vi "uEye_SimpleLive.vi"() -> ()   [LabVIEW 2016]
uses:
  C:/Program Files/National Instruments/LabVIEW 2016/instr.lib/IDS/ueye.NET/uEyeDotNet.dll
  Program Files/National Instruments/LabVIEW 2016/instr.lib/IDS/ueye.NET/uEyeDotNet.dll
  System.Windows.Forms
panel:
  in  "Exposure":dbl(slide) min=0.07826829268292683 max=49.96831707317074 step=0.021121951219512197 scale=0.0769533433340476..166.26649730429713
  out "MinFps":i32=8
  out "MaxFps":i32=8
  in  "Framerate":dbl min=3.056022538005872 max=6.160183642413259 step=0.0031285848869551103
  in  "Pixelclock":u16(ring) items=["5", "6", "7", "8", "9", "10", "11", "12", "13", "14", "15", "16", "17", "18", "19", "20", "21", "22", "23", "24", "25", "26", "27", "28", "29", "30", "31", "32", "33", "34", "35", "36", "37", "38", "39", "40", "41", "42"]
  in  "Auto Exposure":bool
  in  "Zoom":u16(ring)=1 items=["4X"=4, "2X"=2, "1X"=1]
  in  "PictureBox":refnum<k24>(container)
  out "Serial Number 2":string
  out "Height 2":i32=8
  out "Width 2":i32=8
  out "Bits/Pixel 2":i32=8
  in  "Camera ID":i32
  out "Serial Number":string
  out "Height":i32=8
  out "Width":i32=8
  out "Bits/Pixel":i32=8
  out "Error Out":errorcluster caption="error"
  in  "Load Parameter":bool
  in  "Exit Camera":bool
  in  "Stop Live":bool
  in  "Start Live":bool
  in  "Init Camera":bool
  # "-"
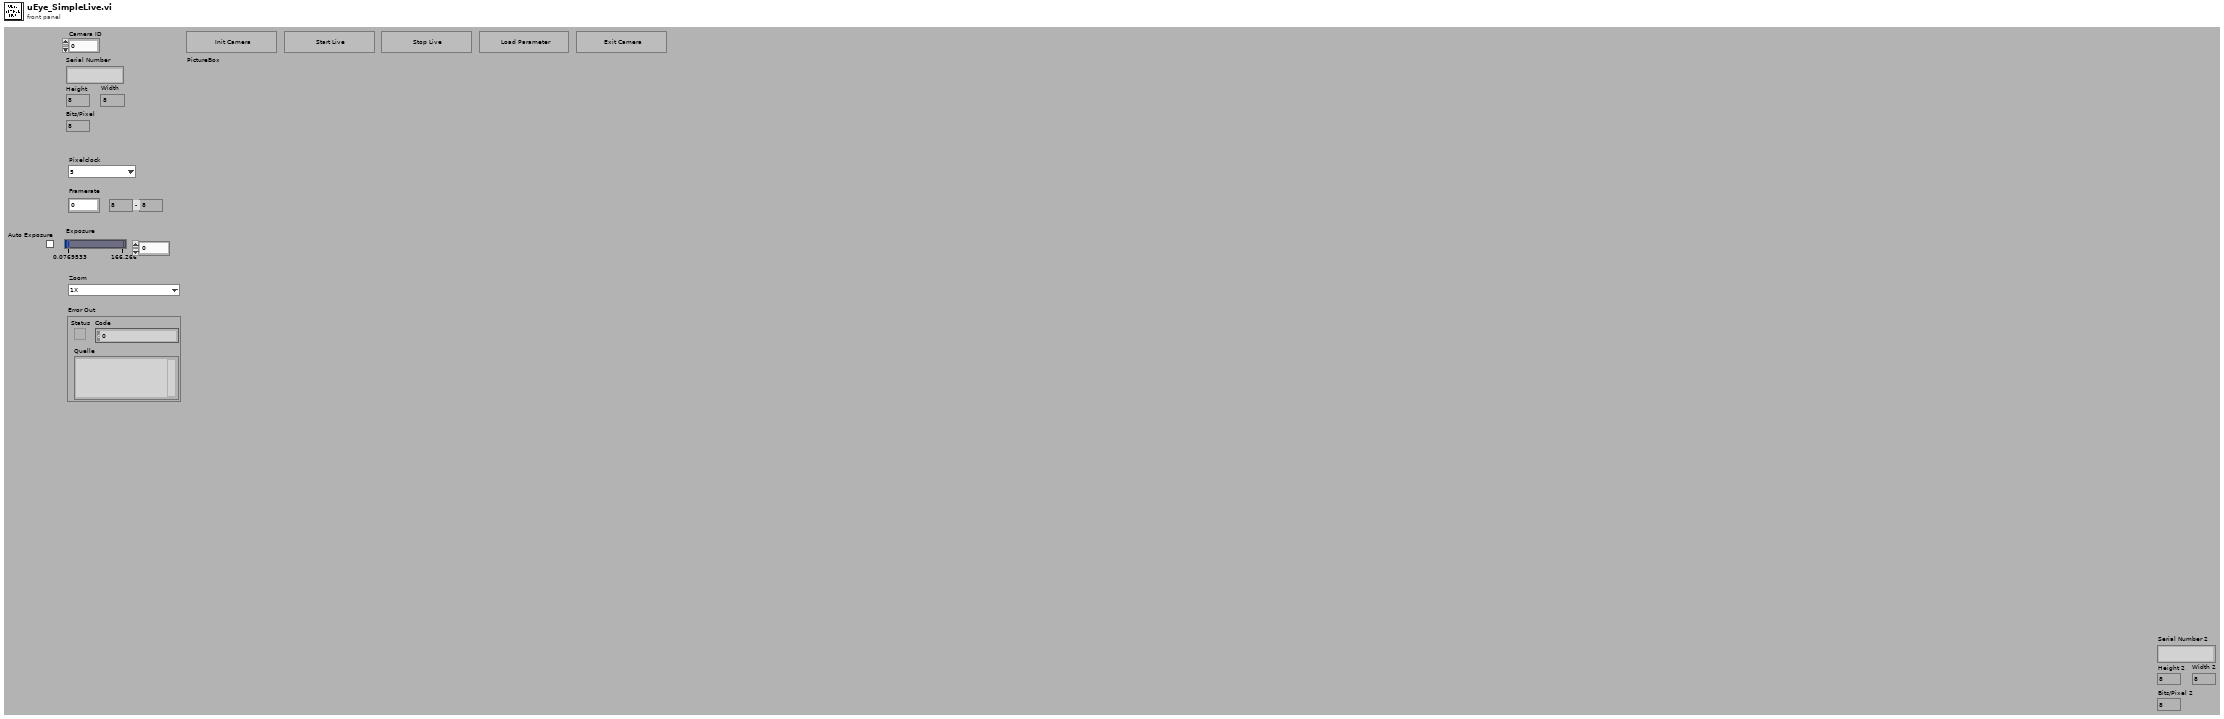
[diagram p1: front panel]
types:
  T1 = enum8{"Enabled", "Disabled", "Disabled and Grayed Out"}
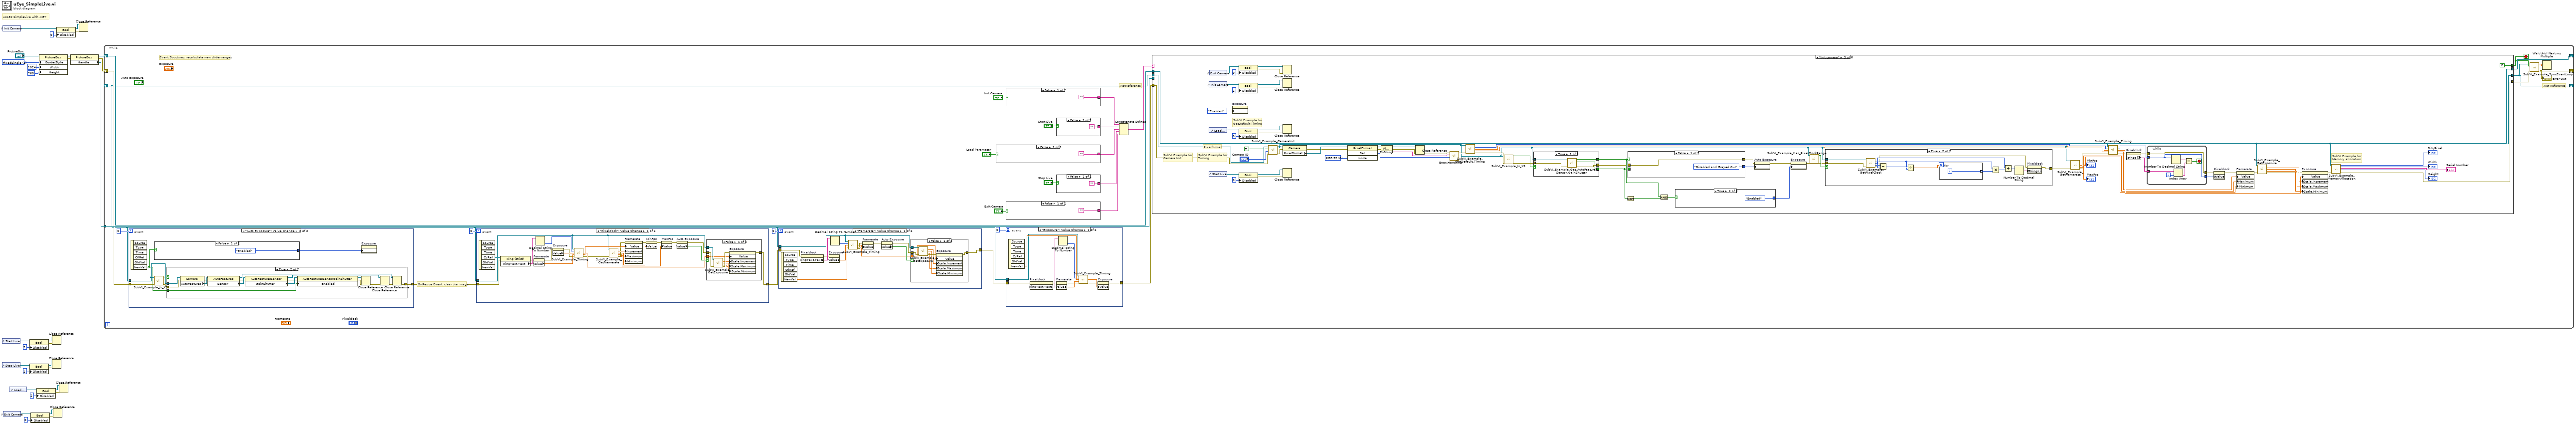
[diagram p0: block diagram]
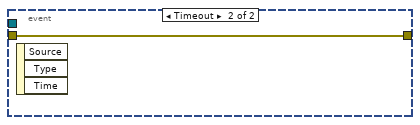
[diagram p2: hidden frame]
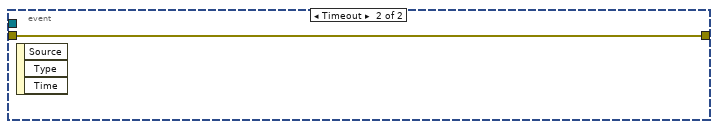
[diagram p4: hidden frame]
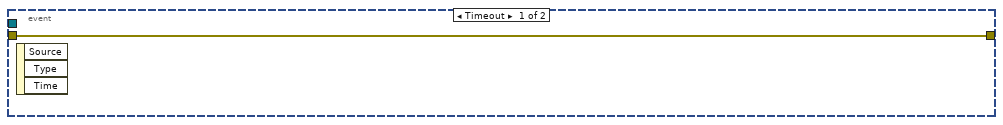
[diagram p5: hidden frame]
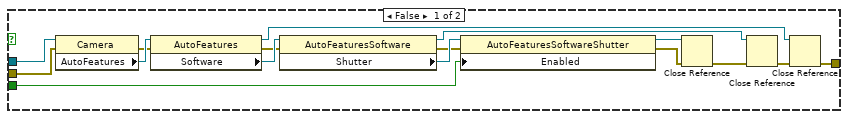
[diagram p6: hidden frame]
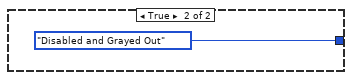
[diagram p7: hidden frame]
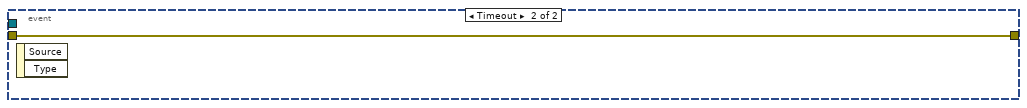
[diagram p9: hidden frame]
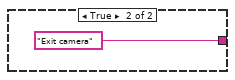
[diagram p10: hidden frame]
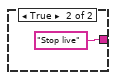
[diagram p11: hidden frame]
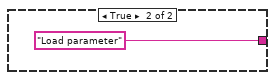
[diagram p12: hidden frame]
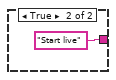
[diagram p13: hidden frame]
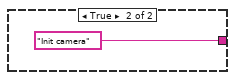
[diagram p14: hidden frame]
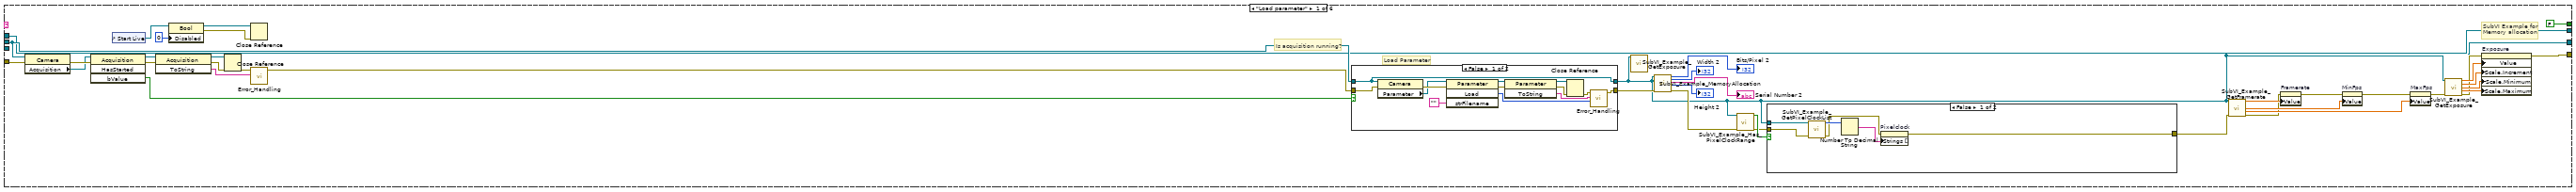
[diagram p15: hidden frame]
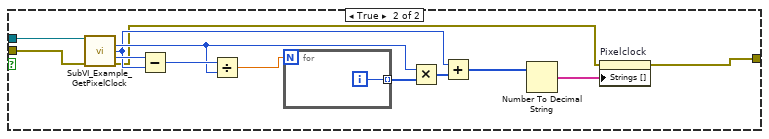
[diagram p16: hidden frame]
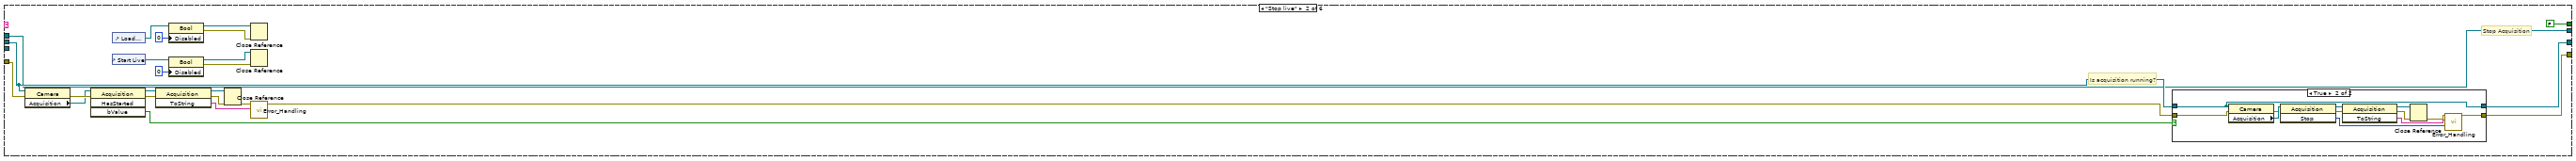
[diagram p18: hidden frame]
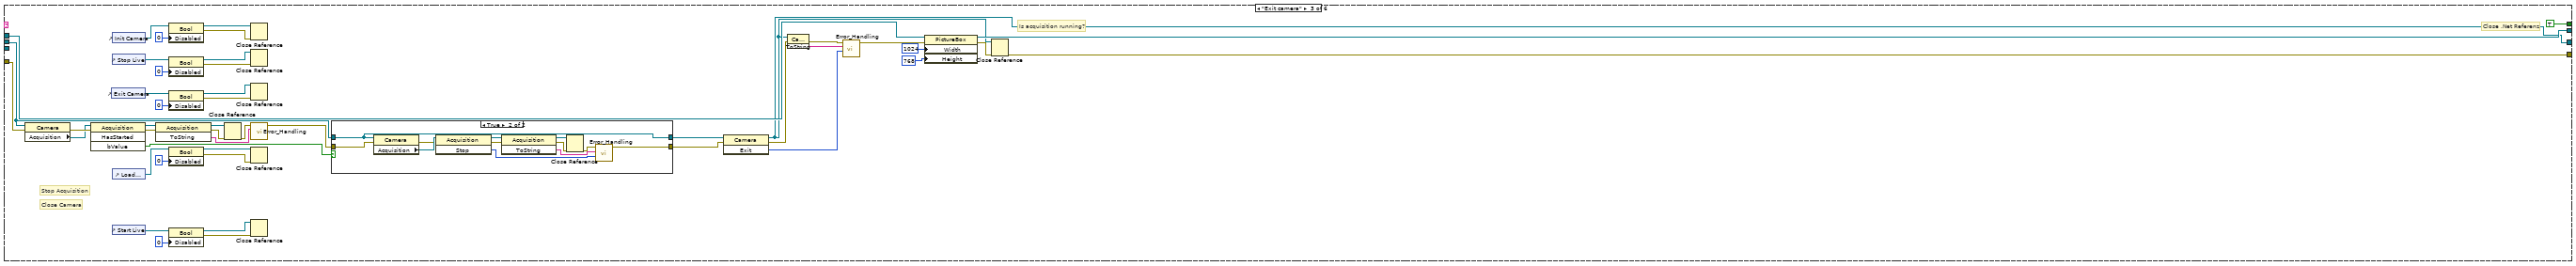
[diagram p20: hidden frame]
diagram:
  w18 = 1 items=["None", "FixedSingle", "Fixed3D"] ("BorderStyle")
  # "uc480 SimpleLive with .NET"
  n1 = control-ref of="Start Live"() -> (w26:refnum<vi>)
  n2 = control-ref of="Stop Live"() -> (w20:refnum<vi>)
  n3 = control-ref of="Init Camera"() -> (w29:refnum<vi>)
  n4 = control-ref of="Exit Camera"() -> (w22:refnum<vi>)
  n5 = control-ref of="Load Parameter"() -> (w21:refnum<vi>)
  n6 = property class="Bool"(reference=w26, "Disabled"=u8 2 ("Deaktiviert")) -> (reference out=w13:refnum<vi>, error out=w12:errorcluster)  [unwired: 1 in]
  n7 = property class="Bool"(reference=w20, "Disabled"=u8 2 ("Deaktiviert")) -> (reference out=w11:refnum<vi>, error out=w10:errorcluster)  [unwired: 1 in]
  n8 = property class="Bool"(reference=w22, "Disabled"=u8 0 ("Deaktiviert")) -> (reference out=w7:refnum<vi>, error out=w6:errorcluster)  [unwired: 1 in]
  n9 = property class="Bool"(reference=w21, "Disabled"=u8 2 ("Deaktiviert")) -> (reference out=w9:refnum<vi>, error out=w8:errorcluster)  [unwired: 1 in]
  n10 = property class="PictureBox"(reference="PictureBox", "BorderStyle"=w18, "Width"=1024, "Height"=768) -> (reference out=w4:refnum<k24>, error out=w5:errorcluster)  [unwired: 1 in]
  n11 = Close Reference(reference=w13, error in (no error)=w12) -> ()  [unwired: 1 out]
  n12 = Close Reference(reference=w11, error in (no error)=w10) -> ()  [unwired: 1 out]
  n13 = Close Reference(reference=w7, error in (no error)=w6) -> ()  [unwired: 1 out]
  n14 = property class="Bool"(reference=w29, "Disabled"=u8 0 ("Deaktiviert")) -> (reference out=w15:refnum<vi>, error out=w14:errorcluster)  [unwired: 1 in]
  n15 = Close Reference(reference=w9, error in (no error)=w8) -> ()  [unwired: 1 out]
  n16 = property class="PictureBox"(reference=w4, error in=w5) -> (reference out=w3:refnum<k24>, error out=w2:errorcluster, "Handle"=w1:refnum<k24>)
  n17 = Close Reference(reference=w15, error in (no error)=w14) -> ()  [unwired: 1 out]
  n18 = while {
    shift-right: [w45] -> _
    shift-left: w2 -> [w41]
    shift-right: [w30] -> _
    shift-left: _ -> [w35]
    shift-right: [w44] -> _
    shift-left: w3 -> [w40]
    tunnel: w1 -> [w43]
    stop <- w31 stop-if-true
    # "OnResize Event, clear the image"
    # "Event Structures, recalculate new slider ranges"
    # ".NetReference"
    # ".Net Reference"
    n19 = event shown="[1] \"Auto Exposure\": Value Change" {
      selector: _ -> [_ _]
      dyn-events: _ -> [_ _]
      timeout: 0 -> [_ _]
      tunnel: w41 -> [w95 w102]
      tunnel: w35 -> [_ w100]
      tunnel: [w95 w97] -> w39
      event Timeout {
        n20 = event-data() -> ()  [unwired: 1 in, 3 out]
      }
      event "Auto Exposure": Value Change {
        n21 = event-data() -> ("NewVal"=w99:bool)  [unwired: 1 in, 5 out]
        n22 = case shown="False" w99 {
          tunnel: [T1."Enabled" ("Deaktiviert") T1."Disabled and Grayed Out" ("Deaktiviert")] -> w96
          frame False {
          }
          frame True {
          }
        }
        n23 = call "SubVI_Example_Is_XS.vi"("Error In"=w102, ".NET (Reference)"=w100) -> ("Error Out"=w101:errorcluster, "IsXS"=w98:bool)  [unwired: 7 in, 1 out]
        n24 = case shown="True" w98 {
          tunnel: w101 -> [w106 w133]
          tunnel: [w103 w119] -> w97
          tunnel: w100 -> [w105 w134]
          tunnel: w99 -> [w104 w126]
          frame False {
            n25 = property on="Eigenschaftsknoten" class="Camera"(reference=w105, error in=w106) -> (error out=w117:errorcluster, "AutoFeatures"=w118:refnum<k24>)  [unwired: 1 out]
            n26 = property on="Eigenschaftsknoten" class="AutoFeatures"(reference=w118, error in=w117) -> (reference out=w107:refnum<k24>, error out=w115:errorcluster, "Software"=w116:refnum<k24>)
            n27 = property on="Eigenschaftsknoten" class="AutoFeaturesSoftware"(reference=w116, error in=w115) -> (reference out=w110:refnum<k24>, error out=w113:errorcluster, "Shutter"=w114:refnum<k24>)
            n28 = property on="Eigenschaftsknoten" class="AutoFeaturesSoftwareShutter"(reference=w114, error in=w113, "Enabled"=w104) -> (reference out=w112:refnum<k24>, error out=w111:errorcluster)
            n29 = Close Reference(reference=w112, error in (no error)=w111) -> (error out=w109:errorcluster)
            n30 = Close Reference(reference=w110, error in (no error)=w109) -> (error out=w108:errorcluster)
            n31 = Close Reference(reference=w107, error in (no error)=w108) -> (error out=w103:errorcluster)
          }
          frame True {
            n32 = property on="Eigenschaftsknoten" class="Camera"(reference=w134, error in=w133) -> (error out=w131:errorcluster, "AutoFeatures"=w132:refnum<k24>)  [unwired: 1 out]
            n33 = property on="Eigenschaftsknoten" class="AutoFeatures"(reference=w132, error in=w131) -> (reference out=w120:refnum<k24>, error out=w129:errorcluster, "Sensor"=w130:refnum<k24>)
            n34 = property on="Eigenschaftsknoten" class="AutoFeaturesSensor"(reference=w130, error in=w129) -> (reference out=w123:refnum<k24>, error out=w127:errorcluster, "GainShutter"=w128:refnum<k24>)
            n35 = property on="Eigenschaftsknoten" class="AutoFeaturesSensorGainShutter"(reference=w128, error in=w127, "Enabled"=w126) -> (reference out=w125:refnum<k24>, error out=w124:errorcluster)
            n36 = Close Reference(reference=w125, error in (no error)=w124) -> (error out=w122:errorcluster)
            n37 = Close Reference(reference=w123, error in (no error)=w122) -> (error out=w121:errorcluster)
            n38 = Close Reference(reference=w120, error in (no error)=w121) -> (error out=w119:errorcluster)
          }
        }
        n39 = property on="Exposure" class="Slide (strict)"("DisabledEnum"=w96) -> ()  [unwired: 2 in, 2 out]
      }
    }
    n40 = event shown="[0] \"Pixelclock\": Value Change" {
      selector: _ -> [_ _]
      dyn-events: _ -> [_ _]
      timeout: 0 -> [_ _]
      tunnel: w35 -> [w149 _]
      tunnel: w39 -> [w141 w169]
      tunnel: [w146 w169] -> w38
      event "Pixelclock": Value Change {
        n41 = event-data() -> ("CtlRef"=w144:refnum<vi>)  [unwired: 1 in, 5 out]
        n42 = property class="Ring (strict)"(reference=w144, error in=w141) -> (error out=w140:errorcluster, "RingText.Text"=w143:string)  [unwired: 1 out]
        n43 = property on="Framerate" class="DigNum (strict)"(error in=w140) -> (error out=w139:errorcluster, "Value"=w159:dbl)  [unwired: 1 in, 1 out]
        n44 = Decimal String To Number(string=w143) -> (number=w142:i32)  [unwired: 2 in, 1 out]
        n45 = property on="Exposure" class="Slide (strict)"(error in=w139) -> (error out=w138:errorcluster, "Value"=w158:dbl)  [unwired: 1 in, 1 out]
        n46 = call "SubVI_Example_Timing.vi"(".NET (Reference)"=w149, "Pixelclock"=w142, "Exposure time"=w158, "Framerate"=w159, "Error In"=w138) -> ("Exposure time"=w145:dbl, "Framerate"=w156:dbl, "Error Out"=w137:errorcluster)  [unwired: 7 in, 1 out]
        n47 = call "SubVI_Example_GetFramerate.vi"(".NET (Reference)"=w149, "Error In"=w137) -> ("Inc"=w157:dbl, "Min"=w154:dbl, "Max"=w153:dbl, "error out"=w155:errorcluster)  [unwired: 9 in, 1 out]
        n48 = property on="Framerate" class="DigNum (strict)"(error in=w155, "Value"=w156, "Increment"=w157, "Maximum"=w153, "Minimum"=w154) -> (error out=w152:errorcluster)  [unwired: 1 in, 1 out]
        n49 = property on="MinFps" class="DigNum (strict)"(error in=w152, "Value"=w154) -> (error out=w151:errorcluster)  [unwired: 1 in, 1 out]
        n50 = property on="MaxFps" class="DigNum (strict)"(error in=w151, "Value"=w153) -> (error out=w148:errorcluster)  [unwired: 1 in, 1 out]
        n51 = property on="Auto Exposure" class="Bool (strict)"(error in=w148) -> (error out=w147:errorcluster, "Value"=w150:bool)  [unwired: 1 in, 1 out]
        n52 = case shown="False" w150 {
          tunnel: w149 -> [w167 _]
          tunnel: w147 -> [w166 w168]
          tunnel: [w164 w168] -> w146
          tunnel: w145 -> [w160 _]
          frame False {
            n53 = call "SubVI_Example_GetExposure.vi"(".NET (Reference)"=w167, "Error In"=w166) -> ("Inc"=w161:dbl, "Min"=w163:dbl, "Max"=w162:dbl, "Error out"=w165:errorcluster)  [unwired: 9 in, 1 out]
            n54 = property on="Exposure" class="Slide (strict)"(error in=w165, "Value"=w160, "Scale.Increment"=w161, "Scale.Maximum"=w162, "Scale.Minimum"=w163) -> (error out=w164:errorcluster)  [unwired: 1 in, 1 out]
          }
          frame True {
          }
        }
      }
      event Timeout {
        n55 = event-data() -> ()  [unwired: 1 in, 2 out]
      }
    }
    n56 = event shown="[0] \"Framerate\": Value Change" {
      selector: _ -> [_ _]
      dyn-events: _ -> [_ _]
      timeout: 0 -> [_ _]
      tunnel: w38 -> [w72 w94]
      tunnel: w35 -> [w76 _]
      tunnel: [w77 w94] -> w34
      event "Framerate": Value Change {
        n57 = event-data() -> ("NewVal"=w84:dbl)  [unwired: 1 in, 5 out]
        n58 = property on="Pixelclock" class="Ring (strict)"(error in=w72) -> (error out=w71:errorcluster, "RingText.Text"=w74:string)  [unwired: 1 in, 1 out]
        n59 = property on="Exposure" class="Slide (strict)"(error in=w71) -> ("Value"=w83:dbl)  [unwired: 1 in, 2 out]
        n60 = Decimal String To Number(string=w74) -> (number=w73:i32)  [unwired: 2 in, 1 out]
        n61 = call "SubVI_Example_Timing.vi"(".NET (Reference)"=w76, "Pixelclock"=w73, "Exposure time"=w83, "Framerate"=w84) -> ("Exposure time"=w75:dbl, "Framerate"=w82:dbl, "Error Out"=w80:errorcluster)  [unwired: 8 in, 1 out]
        n62 = property on="Framerate" class="DigNum (strict)"(error in=w80, "Value"=w82) -> (error out=w79:errorcluster)  [unwired: 1 in, 1 out]
        n63 = property on="Auto Exposure" class="Bool (strict)"(error in=w79) -> (error out=w78:errorcluster, "Value"=w81:bool)  [unwired: 1 in, 1 out]
        n64 = case shown="False" w81 {
          tunnel: w78 -> [w92 w93]
          tunnel: [w90 w93] -> w77
          tunnel: w76 -> [w89 _]
          tunnel: w75 -> [w85 _]
          frame False {
            n65 = call "SubVI_Example_GetExposure.vi"(".NET (Reference)"=w89, "Error In"=w92) -> ("Inc"=w87:dbl, "Min"=w88:dbl, "Max"=w86:dbl, "Error out"=w91:errorcluster)  [unwired: 9 in, 1 out]
            n66 = property on="Exposure" class="Slide (strict)"(error in=w91, "Value"=w85, "Scale.Increment"=w87, "Scale.Maximum"=w86, "Scale.Minimum"=w88) -> (error out=w90:errorcluster)  [unwired: 1 in, 1 out]
          }
          frame True {
          }
        }
      }
      event Timeout {
        n67 = event-data() -> ()  [unwired: 1 in, 3 out]
      }
    }
    n68 = case shown="False" "Load Parameter" {
      tunnel: ["" "Load parameter"] -> w52
      frame False {
      }
      frame True {
      }
    }
    n69 = case shown="False" "Init Camera" {
      tunnel: ["" "Init camera"] -> w56
      frame False {
      }
      frame True {
      }
    }
    n70 = case shown="False" "Exit Camera" {
      tunnel: ["" "Exit camera"] -> w48
      frame False {
      }
      frame True {
      }
    }
    n71 = event shown="[0] \"Exposure\": Value Change" {
      selector: _ -> [_ _]
      dyn-events: _ -> [_ _]
      timeout: 0 -> [_ _]
      tunnel: w35 -> [w65 _]
      tunnel: w34 -> [w61 w70]
      tunnel: [w66 w70] -> w33
      event "Exposure": Value Change {
        n72 = event-data() -> ("NewVal"=w69:dbl)  [unwired: 1 in, 5 out]
        n73 = property on="Pixelclock" class="Ring (strict)"(error in=w61) -> (error out=w60:errorcluster, "RingText.Text"=w63:string)  [unwired: 1 in, 1 out]
        n74 = property on="Framerate" class="DigNum (strict)"(error in=w60) -> (error out=w59:errorcluster, "Value"=w68:dbl)  [unwired: 1 in, 1 out]
        n75 = Decimal String To Number(string=w63) -> (number=w62:i32)  [unwired: 2 in, 1 out]
        n76 = call "SubVI_Example_Timing.vi"(".NET (Reference)"=w65, "Pixelclock"=w62, "Exposure time"=w69, "Framerate"=w68, "Error In"=w59) -> ("Exposure time"=w67:dbl, "Error Out"=w64:errorcluster)  [unwired: 7 in, 2 out]
        n77 = property on="Exposure" class="Slide (strict)"(error in=w64, "Value"=w67) -> (error out=w66:errorcluster)  [unwired: 1 in, 1 out]
      }
      event Timeout {
        n78 = event-data() -> ()  [unwired: 1 in, 3 out]
      }
    }
    n79 = case shown="False" "Start Live" {
      tunnel: ["" "Start live"] -> w55
      frame False {
      }
      frame True {
      }
    }
    n80 = case shown="False" "Stop Live" {
      tunnel: ["" "Stop live"] -> w51
      frame False {
      }
      frame True {
      }
    }
    n81 = Concatenate Strings(w56, w55, w52, w51, w48) -> (w54:string)
    n82 = case shown="\"Init camera\"" w54 {
      tunnel: w35 -> [w211 w271 w326 w360 w482 w552]
      tunnel: w33 -> [w214 w272 w327 w361 w481 w553]
      tunnel: [w181 w270 w335 w358 w451 w550] -> w47
      tunnel: [FALSE FALSE TRUE FALSE FALSE FALSE] -> w31
      tunnel: w40 -> [w203 w264 w306 w366 w463 w543]
      tunnel: [w203 w264 w305 w365 w463 w543] -> w44
      tunnel: w43 -> [_ _ _ w362 _ _]
      tunnel: [w180 w256 w294 w355 w420 w536] -> w30
      frame "Load parameter" {
        # "SubVI Example for \nMemory allocation"
        # "Is acquisition running?"
        # "Load Parameter"
        n83 = property class="Camera"(reference=w211, error in=w214) -> (error out=w219:errorcluster, "Acquisition"=w218:refnum<k24>)  [unwired: 1 out]
        n84 = invoke class="Acquisition" method="HasStarted"(reference=w218, error in=w219) -> (reference out=w215:refnum<k24>, error out=w217:errorcluster, "bValue"=w213:bool)  [unwired: 2 in, 1 out]
        n85 = control-ref of="Start Live"() -> (w205:refnum<vi>)
        n86 = invoke class="Acquisition" method="ToString"(reference=w215, error in=w217) -> (reference out=w200:refnum<k24>, error out=w199:errorcluster, "ToString"=w216:string)  [unwired: 1 in]
        n87 = property class="Bool"(reference=w205, "Disabled"=u8 0 ("Deaktiviert")) -> (reference out=w202:refnum<vi>, error out=w201:errorcluster)  [unwired: 1 in]
        n88 = Close Reference(reference=w200, error in (no error)=w199) -> (error out=w198:errorcluster)
        n89 = Close Reference(reference=w202, error in (no error)=w201) -> ()  [unwired: 1 out]
        n90 = call "Error_Handling.vi"("Error String"=w216, "Error In"=w198) -> ("Error Out"=w212:errorcluster)  [unwired: 9 in]
        n91 = case shown="False" w213 {
          tunnel: w212 -> [w247 w254]
          tunnel: w211 -> [w245 w255]
          tunnel: [w246 w254] -> w206
          tunnel: [w245 w255] -> w180
          frame False {
            n92 = property class="Camera"(reference=w245, error in=w247) -> (error out=w249:errorcluster, "Parameter"=w248:refnum<k24>)  [unwired: 1 out]
            n93 = invoke class="Parameter" method="Load"(reference=w248, error in=w249, "strFilename"="") -> (reference out=w251:refnum<k24>, error out=w252:errorcluster, "Load"=w244:i32)  [unwired: 1 in, 1 out]
            n94 = invoke class="Parameter" method="ToString"(reference=w251, error in=w252) -> (reference out=w241:refnum<k24>, error out=w243:errorcluster, "ToString"=w253:string)  [unwired: 1 in]
            n95 = Close Reference(reference=w241, error in (no error)=w243) -> (error out=w242:errorcluster)
            n96 = call "Error_Handling.vi"("Error Code"=w244, "Error String"=w253, "Error In"=w242) -> ("Error Out"=w246:errorcluster)  [unwired: 8 in]
          }
          frame True {
          }
        }
        n97 = call "SubVI_Example_GetExposure.vi"(".NET (Reference)"=w180) -> ()  [unwired: 10 in, 5 out]
        n98 = call "SubVI_Example_MemoryAllocation.vi"(".NET (Reference)"=w180, "Error In"=w206) -> ("Bits/Pixel 2"=→"Bits/Pixel 2":i32, "Width"=→"Width 2":i32, "Serial Number"=→"Serial Number 2":string, "Height"=→"Height 2":i32, "Error Out"=w197:errorcluster)  [unwired: 13 in]
        n99 = call "SubVI_Example_Has_PixelClockRange.vi"(".NET (Reference)"=w180, "error in (no error)"=w197) -> ("Boolean"=w196:bool, "error out"=w195:errorcluster)  [unwired: 16 in]
        n100 = case shown="False" w196 {
          tunnel: w195 -> [w226 w239]
          tunnel: w180 -> [w225 w238]
          tunnel: [w221 w227] -> w194
          frame False {
            n101 = call "SubVI_Example_GetPixelClockList.vi"("error in (no error)"=w226, ".NET (Reference)"=w225) -> ("error out"=w222:errorcluster, "List"=w224:i32[])  [unwired: 7 in, 1 out]
            n102 = Number To Decimal String(number=w224) -> (decimal integer string=w223:string[])  [unwired: 1 in]
            n103 = property on="Pixelclock" class="Ring (strict)"(error in=w222, "Strings []"=w223) -> (error out=w221:errorcluster)  [unwired: 1 in, 1 out]
          }
          frame True {
            n104 = call "SubVI_Example_GetPixelClock.vi"(".NET (Reference)"=w238, "Error In"=w239) -> ("Inc"=w233:i32, "Min"=w231:i32, "Max"=w237:i32, "error out"=w228:errorcluster)  [unwired: 9 in, 1 out]
            n105 = Subtract(x=w237, y=w231) -> (x-y=w236:i32)
            n106 = Divide(x=w236, y=w233) -> (x/y=w235:dbl)
            n107 = for {
              N: w235 -> [_]
              tunnel: [w240] -> w234 mode=indexing
              i -> [w240]
            }
            n108 = Multiply(x=w233, y=w234) -> (x*y=w232:i32[])
            n109 = Add(x=w231, y=w232) -> (x+y=w230:i32[])
            n110 = Number To Decimal String(number=w230) -> (decimal integer string=w229:string[])  [unwired: 1 in]
            n111 = property on="Pixelclock" class="Ring (strict)"(error in=w228, "Strings []"=w229) -> (error out=w227:errorcluster)  [unwired: 1 in, 1 out]
          }
        }
        n112 = call "SubVI_Example_GetFramerate.vi"(".NET (Reference)"=w180, "Error In"=w194) -> ("Framerate"=w193:dbl, "Min"=w192:dbl, "Max"=w191:dbl, "error out"=w190:errorcluster)  [unwired: 9 in, 1 out]
        n113 = property on="Framerate" class="DigNum (strict)"(error in=w190, "Value"=w193) -> (error out=w189:errorcluster)  [unwired: 1 in, 1 out]
        n114 = property on="MinFps" class="DigNum (strict)"(error in=w189, "Value"=w192) -> (error out=w188:errorcluster)  [unwired: 1 in, 1 out]
        n115 = property on="MaxFps" class="DigNum (strict)"(error in=w188, "Value"=w191) -> (error out=w187:errorcluster)  [unwired: 1 in, 1 out]
        n116 = call "SubVI_Example_GetExposure.vi"(".NET (Reference)"=w180, "Error In"=w187) -> ("Exposure"=w186:dbl, "Inc"=w184:dbl, "Min"=w183:dbl, "Max"=w185:dbl, "Error out"=w182:errorcluster)  [unwired: 9 in]
        n117 = property on="Exposure" class="Slide (strict)"(error in=w182, "Value"=w186, "Scale.Increment"=w184, "Scale.Minimum"=w183, "Scale.Maximum"=w185) -> (error out=w181:errorcluster)  [unwired: 1 in, 1 out]
      }
      frame "Stop live" {
        # "Is acquisition running?"
        # "Stop Acquisition"
        n118 = property class="Camera"(reference=w271, error in=w272) -> (error out=w279:errorcluster, "Acquisition"=w278:refnum<k24>)  [unwired: 1 out]
        n119 = invoke class="Acquisition" method="HasStarted"(reference=w278, error in=w279) -> (reference out=w273:refnum<k24>, error out=w275:errorcluster, "bValue"=w277:bool)  [unwired: 2 in, 1 out]
        n120 = control-ref of="Load Parameter"() -> (w268:refnum<vi>)
        n121 = control-ref of="Start Live"() -> (w265:refnum<vi>)
        n122 = invoke class="Acquisition" method="ToString"(reference=w273, error in=w275) -> (reference out=w257:refnum<k24>, error out=w259:errorcluster, "ToString"=w274:string)  [unwired: 1 in]
        n123 = property class="Bool"(reference=w268, "Disabled"=u8 0 ("Deaktiviert")) -> (reference out=w263:refnum<vi>, error out=w262:errorcluster)  [unwired: 1 in]
        n124 = property class="Bool"(reference=w265, "Disabled"=u8 0 ("Deaktiviert")) -> (reference out=w261:refnum<vi>, error out=w260:errorcluster)  [unwired: 1 in]
        n125 = Close Reference(reference=w257, error in (no error)=w259) -> (error out=w258:errorcluster)
        n126 = Close Reference(reference=w263, error in (no error)=w262) -> ()  [unwired: 1 out]
        n127 = Close Reference(reference=w261, error in (no error)=w260) -> ()  [unwired: 1 out]
        n128 = call "Error_Handling.vi"("Error String"=w274, "Error In"=w258) -> ("Error Out"=w276:errorcluster)  [unwired: 9 in]
        n129 = case shown="True" w277 {
          tunnel: [w281 w292] -> w270
          tunnel: w276 -> [w281 w293]
          tunnel: w271 -> [w280 w285]
          tunnel: [w280 w285] -> w256
          frame False {
          }
          frame True {
            n130 = property class="Camera"(reference=w285, error in=w293) -> (error out=w289:errorcluster, "Acquisition"=w290:refnum<k24>)  [unwired: 1 out]
            n131 = invoke class="Acquisition" method="Stop"(reference=w290, error in=w289) -> (reference out=w287:refnum<k24>, error out=w288:errorcluster, "Stop"=w286:i32)  [unwired: 1 in]
            n132 = invoke class="Acquisition" method="ToString"(reference=w287, error in=w288) -> (reference out=w282:refnum<k24>, error out=w284:errorcluster, "ToString"=w291:string)  [unwired: 1 in]
            n133 = Close Reference(reference=w282, error in (no error)=w284) -> (error out=w283:errorcluster)
            n134 = call "Error_Handling.vi"("Error Code"=w286, "Error String"=w291, "Error In"=w283) -> ("Error Out"=w292:errorcluster)  [unwired: 8 in]
          }
        }
      }
      frame "Exit camera" {
        # "Close .Net Referenz"
        # "Is acquisition running?"
        # "Stop Acquisition"
        # "Close Camera"
        n135 = property class="Camera"(reference=w326, error in=w327) -> (error out=w334:errorcluster, "Acquisition"=w333:refnum<k24>)  [unwired: 1 out]
        n136 = invoke class="Acquisition" method="HasStarted"(reference=w333, error in=w334) -> (reference out=w328:refnum<k24>, error out=w330:errorcluster, "bValue"=w332:bool)  [unwired: 2 in, 1 out]
        n137 = control-ref of="Exit Camera"() -> (w314:refnum<vi>)
        n138 = control-ref of="Init Camera"() -> (w318:refnum<vi>)
        n139 = control-ref of="Stop Live"() -> (w315:refnum<vi>)
        n140 = control-ref of="Load Parameter"() -> (w316:refnum<vi>)
        n141 = control-ref of="Start Live"() -> (w317:refnum<vi>)
        n142 = invoke class="Acquisition" method="ToString"(reference=w328, error in=w330) -> (reference out=w311:refnum<k24>, error out=w313:errorcluster, "ToString"=w329:string)  [unwired: 1 in]
        n143 = property class="Bool"(reference=w318, "Disabled"=u8 0 ("Deaktiviert")) -> (reference out=w296:refnum<vi>, error out=w295:errorcluster)  [unwired: 1 in]
        n144 = property class="Bool"(reference=w315, "Disabled"=u8 0 ("Deaktiviert")) -> (reference out=w302:refnum<vi>, error out=w301:errorcluster)  [unwired: 1 in]
        n145 = property class="Bool"(reference=w314, "Disabled"=u8 0 ("Deaktiviert")) -> (reference out=w304:refnum<vi>, error out=w303:errorcluster)  [unwired: 1 in]
        n146 = property class="Bool"(reference=w316, "Disabled"=u8 0 ("Deaktiviert")) -> (reference out=w300:refnum<vi>, error out=w299:errorcluster)  [unwired: 1 in]
        n147 = property class="Bool"(reference=w317, "Disabled"=u8 0 ("Deaktiviert")) -> (reference out=w298:refnum<vi>, error out=w297:errorcluster)  [unwired: 1 in]
        n148 = Close Reference ("Close Referenz")(reference=w311, error in (no error)=w313) -> (error out=w312:errorcluster)
        n149 = Close Reference(reference=w296, error in (no error)=w295) -> ()  [unwired: 1 out]
        n150 = Close Reference(reference=w302, error in (no error)=w301) -> ()  [unwired: 1 out]
        n151 = Close Reference(reference=w304, error in (no error)=w303) -> ()  [unwired: 1 out]
        n152 = call "Error_Handling.vi"("Error String"=w329, "Error In"=w312) -> ("Error Out"=w331:errorcluster)  [unwired: 9 in]
        n153 = Close Reference(reference=w300, error in (no error)=w299) -> ()  [unwired: 1 out]
        n154 = Close Reference(reference=w298, error in (no error)=w297) -> ()  [unwired: 1 out]
        n155 = case shown="True" w332 {
          tunnel: [w342 w353] -> w324
          tunnel: w331 -> [w342 w354]
          tunnel: w326 -> [w341 w346]
          tunnel: [w341 w346] -> w325
          frame False {
          }
          frame True {
            n156 = property class="Camera"(reference=w346, error in=w354) -> (error out=w350:errorcluster, "Acquisition"=w351:refnum<k24>)  [unwired: 1 out]
            n157 = invoke class="Acquisition" method="Stop"(reference=w351, error in=w350) -> (reference out=w348:refnum<k24>, error out=w349:errorcluster, "Stop"=w347:i32)  [unwired: 1 in]
            n158 = invoke class="Acquisition" method="ToString"(reference=w348, error in=w349) -> (reference out=w343:refnum<k24>, error out=w345:errorcluster, "ToString"=w352:string)  [unwired: 1 in]
            n159 = Close Reference ("Close Referenz")(reference=w343, error in (no error)=w345) -> (error out=w344:errorcluster)
            n160 = call "Error_Handling.vi"("Error Code"=w347, "Error String"=w352, "Error In"=w344) -> ("Error Out"=w353:errorcluster)  [unwired: 8 in]
          }
        }
        n161 = invoke class="Camera" method="Exit"(reference=w325, error in=w324) -> (reference out=w294:refnum<k24>, error out=w337:errorcluster, "Exit"=w336:i32)  [unwired: 1 in]
        n162 = invoke class="Camera" method="ToString"(reference=w294, error in=w337) -> (error out=w338:errorcluster, "ToString"=w339:string)  [unwired: 1 in, 1 out]
        n163 = call "Error_Handling.vi"("Error Code"=w336, "Error String"=w339, "Error In"=w338) -> ("Error Out"=w310:errorcluster)  [unwired: 8 in]
        n164 = property class="PictureBox"(reference=w306, error in=w310, "Width"=1024, "Height"=768) -> (reference out=w305:refnum<k24>, error out=w309:errorcluster)
        n165 = Close Reference ("Close Referenz")(reference=w294, error in (no error)=w309) -> (error out=w335:errorcluster)
      }
      frame Default {
        # "Has acquisition started?"
        n166 = property class="Camera"(reference=w360, error in=w361) -> (reference out=w367:refnum<k24>, error out=w376:errorcluster, "Acquisition"=w375:refnum<k24>)
        n167 = invoke class="Acquisition" method="HasStarted"(reference=w375, error in=w376) -> (reference out=w364:refnum<k24>, error out=w372:errorcluster, "HasStarted"=w371:i32, "bValue"=w363:bool)  [unwired: 2 in]
        n168 = invoke class="Acquisition" method="ToString"(reference=w364, error in=w372) -> (reference out=w368:refnum<k24>, error out=w374:errorcluster, "ToString"=w373:string)  [unwired: 1 in]
        n169 = call "Error_Handling.vi"("Error Code"=w371, "Error String"=w373, "Error In"=w374) -> ("Error Out"=w370:errorcluster)  [unwired: 8 in]
        n170 = Close Reference(reference=w368, error in (no error)=w370) -> (error out=w369:errorcluster)
        n171 = case "Show Image" shown="True" w363 {
          tunnel: [w386 w387] -> w356
          tunnel: w369 -> [w386 w403]
          tunnel: w367 -> [w385 w402]
          tunnel: [w385 w407] -> w355
          tunnel: w366 -> [w384 w404]
          tunnel: [w384 w389] -> w365
          tunnel: w362 -> [_ w388]
          frame False {
          }
          frame True {
            n172 = local read "Height"() -> (w400:i32)
            n173 = local read "Width"() -> (w396:i32)
            n174 = Divide(x=w396, y="Zoom") -> (x/y=w398:dbl)
            n175 = Divide(x=w400, y="Zoom") -> (x/y=w401:dbl)
            n176 = To Long Integer(number=w398) -> (32bit integer=w397:i32)
            n177 = To Long Integer(number=w401) -> (32bit integer=w399:i32)
            n178 = property class="PictureBox"(reference=w404, error in=w403, "Width"=w397, "Height"=w399) -> (reference out=w389:refnum<k24>, error out=w390:errorcluster)
            n179 = property class="Camera"(reference=w402, error in=w390) -> (reference out=w408:refnum<k24>, error out=w411:errorcluster, "Memory"=w412:refnum<k24>)
            n180 = invoke class="Memory" method="GetActive"(reference=w412, error in=w411) -> (reference out=w391:refnum<k24>, error out=w392:errorcluster, "s32MemId"=w406:i32)  [unwired: 2 in, 1 out]
            n181 = property class="Camera"(reference=w408, error in=w392) -> (reference out=w407:refnum<k24>, error out=w405:errorcluster, "Display"=w410:refnum<k24>)
            n182 = invoke class="Display" method="Render"(reference=w410, error in=w405, "memID"=w406, "windowHandle"=w388) -> (reference out=w409:refnum<k24>, error out=w394:errorcluster)  [unwired: 1 in, 3 out]
            n183 = Close Reference(reference=w409, error in (no error)=w394) -> (error out=w393:errorcluster)
            n184 = Close Reference(reference=w391, error in (no error)=w393) -> (error out=w387:errorcluster)
          }
        }
        n185 = property on="Auto Exposure" class="Bool (strict)"(error in=w356) -> (error out=w357:errorcluster, "Value"=w359:bool)  [unwired: 1 in, 1 out]
        n186 = case shown="True" w359 {
          tunnel: w357 -> [w378 w383]
          tunnel: [w378 w379] -> w358
          tunnel: w355 -> [_ w381]
          frame False {
          }
          frame True {
            n187 = call "SubVI_Example_GetExposure.vi"(".NET (Reference)"=w381, "Error In"=w383) -> ("Exposure"=w382:dbl, "Error out"=w380:errorcluster)  [unwired: 9 in, 3 out]
            n188 = property on="Exposure" class="Slide (strict)"(error in=w380, "Value"=w382) -> (error out=w379:errorcluster)  [unwired: 1 in, 1 out]
          }
        }
      }
      frame "Init camera" {
        w490 = 0 items=["RGB 32"=0, "RGB 24"=1, "Y8 Monochrom"=6] ("Mode")
        # "SubVI Example for \nGetDefault Timing"
        # "SubVI Example for \nMemory allocation"
        # "SubVI Example for \nTiming"
        # "SubVI Example for \nCamera Init"
        # "Pixelformat"
        n189 = control-ref of="Init Camera"() -> (w470:refnum<vi>)
        n190 = control-ref of="Load Parameter"() -> (w466:refnum<vi>)
        n191 = control-ref of="Start Live"() -> (w468:refnum<vi>)
        n192 = control-ref of="Exit Camera"() -> (w464:refnum<vi>)
        n193 = property on="Exposure" class="Slide (strict)"("DisabledEnum"=T1."Enabled" ("Disabled")) -> ()  [unwired: 2 in, 2 out]
        n194 = property class="Bool"(reference=w464, "Disabled"=u8 0 ("Deaktiviert")) -> (reference out=w456:refnum<vi>, error out=w455:errorcluster)  [unwired: 1 in]
        n195 = property class="Bool"(reference=w470, "Disabled"=u8 2 ("Deaktiviert")) -> (reference out=w462:refnum<vi>, error out=w461:errorcluster)  [unwired: 1 in]
        n196 = property class="Bool"(reference=w466, "Disabled"=u8 0 ("Deaktiviert")) -> (reference out=w458:refnum<vi>, error out=w457:errorcluster)  [unwired: 1 in]
        n197 = property class="Bool"(reference=w468, "Disabled"=u8 0 ("Deaktiviert")) -> (reference out=w460:refnum<vi>, error out=w459:errorcluster)  [unwired: 1 in]
        n198 = call "SubVI_Example_CameraInit.vi"("Error In"=w481, "Camera ID"="Camera ID", "Init Camera Flag"=TRUE, ".NET (Reference)"=w482) -> ("Error Out"=w487:errorcluster, ".NET (Reference)"=w420:refnum<k24>)  [unwired: 6 in]
        n199 = Close Reference(reference=w456, error in (no error)=w455) -> ()  [unwired: 1 out]
        n200 = Close Reference(reference=w462, error in (no error)=w461) -> ()  [unwired: 1 out]
        n201 = Close Reference(reference=w458, error in (no error)=w457) -> ()  [unwired: 1 out]
        n202 = property on="Property Node" class="Camera"(reference=w420, error in=w487) -> (error out=w488:errorcluster, "PixelFormat"=w489:refnum<k24>)  [unwired: 1 out]
        n203 = Close Reference(reference=w460, error in (no error)=w459) -> ()  [unwired: 1 out]
        n204 = invoke class="PixelFormat" method="Set"(reference=w489, error in=w488, "mode"=w490) -> (reference out=w485:refnum<k24>, error out=w479:errorcluster, "Set"=w484:i32)  [unwired: 1 in, 1 out]
        n205 = invoke class="PixelFormat" method="ToString"(reference=w485, error in=w479) -> (reference out=w452:refnum<k24>, error out=w454:errorcluster, "ToString"=w486:string)  [unwired: 1 in]
        n206 = Close Reference(reference=w452, error in (no error)=w454) -> (error out=w453:errorcluster)
        n207 = call "Error_Handling.vi"("Error Code"=w484, "Error String"=w486, "Error In"=w453) -> ("Error Out"=w448:errorcluster)  [unwired: 8 in]
        n208 = call "SubVI_Example_GetDefault_Timing.vi"(".NET (Reference)"=w420, "Error In"=w448) -> ("Pixelclock"=w474:i32, "Exposure time"=w473:dbl, "Framerate"=w472:dbl, "Error Out"=w446:errorcluster)  [unwired: 10 in]
        n209 = call "SubVI_Example_Is_XS.vi"("Error In"=w446, ".NET (Reference)"=w420) -> ("Error Out"=w447:errorcluster, "IsXS"=w439:bool)  [unwired: 7 in, 1 out]
        n210 = case shown="True" w439 {
          tunnel: w447 -> [w509 w514]
          tunnel: [w508 w513] -> w438
          tunnel: w420 -> [w510 w515]
          tunnel: [w506 w512] -> w442
          tunnel: [w507 w511] -> w440
          frame True {
            n211 = call "SubVI_Example_Get_AutoFeatures_Sensor_GainShutter.vi"("error in (no error)"=w509, ".NET (Reference)"=w510) -> ("error out"=w508:errorcluster, "Enabled"=w507:bool, "Supported"=w506:bool)  [unwired: 6 in]
          }
          frame False {
            n212 = call "SubVI_Example_Get_AutoFeatures_Software_Shutter.vi"("error in (no error)"=w514, ".NET (Reference)"=w515) -> ("error out"=w513:errorcluster, "Enabled"=w511:bool, "Supported"=w512:bool)  [unwired: 7 in]
          }
        }
        n213 = Not(x=w440) -> (.not. x?=w443:bool)
        n214 = case shown="False" w442 {
          tunnel: [T1."Disabled and Grayed Out" ("Deaktiviert") T1."Enabled" ("Deaktiviert")] -> w441
          tunnel: w440 -> [_ w502]
          tunnel: w438 -> [w498 w501]
          tunnel: [w498 w500] -> w437
          frame False {
          }
          frame True {
            n215 = property on="Auto Exposure" class="Bool (strict)"(error in=w501, "Value"=w502) -> (error out=w500:errorcluster)  [unwired: 1 in, 1 out]
          }
        }
        n216 = And(x=w442, y=w443) -> (x .and. y?=w444:bool)
        n217 = case shown="True" w444 {
          tunnel: [T1."Disabled and Grayed Out" ("Disabled") T1."Enabled" ("Disabled")] -> w433
          frame False {
          }
          frame True {
          }
        }
        n218 = property on="Auto Exposure" class="Bool (strict)"(error in=w437, "DisabledEnum"=w441) -> (error out=w432:errorcluster)  [unwired: 1 in, 1 out]
        n219 = property on="Exposure" class="Slide (strict)"(error in=w432, "DisabledEnum"=w433) -> (error out=w431:errorcluster)  [unwired: 1 in, 1 out]
        n220 = call "SubVI_Example_Has_PixelClockRange.vi"(".NET (Reference)"=w420, "error in (no error)"=w431) -> ("Boolean"=w449:bool, "error out"=w436:errorcluster)  [unwired: 16 in]
        n221 = case shown="True" w449 {
          tunnel: w436 -> [w521 w534]
          tunnel: w420 -> [w520 w533]
          tunnel: [w516 w522] -> w435
          frame False {
            n222 = call "SubVI_Example_GetPixelClockList.vi"("error in (no error)"=w521, ".NET (Reference)"=w520) -> ("error out"=w517:errorcluster, "List"=w519:i32[])  [unwired: 7 in, 1 out]
            n223 = Number To Decimal String(number=w519) -> (decimal integer string=w518:string[])  [unwired: 1 in]
            n224 = property on="Pixelclock" class="Ring (strict)"(error in=w517, "Strings []"=w518) -> (error out=w516:errorcluster)  [unwired: 1 in, 1 out]
          }
          frame True {
            n225 = call "SubVI_Example_GetPixelClock.vi"(".NET (Reference)"=w533, "Error In"=w534) -> ("Inc"=w528:i32, "Min"=w526:i32, "Max"=w532:i32, "error out"=w523:errorcluster)  [unwired: 9 in, 1 out]
            n226 = Subtract(x=w532, y=w526) -> (x-y=w531:i32)
            n227 = Divide(x=w531, y=w528) -> (x/y=w530:dbl)
            n228 = for {
              N: w530 -> [_]
              tunnel: [w535] -> w529 mode=indexing
              i -> [w535]
            }
            n229 = Multiply(x=w528, y=w529) -> (x*y=w527:i32[])
            n230 = Add(x=w526, y=w527) -> (x+y=w525:i32[])
            n231 = Number To Decimal String(number=w525) -> (decimal integer string=w524:string[])  [unwired: 1 in]
            n232 = property on="Pixelclock" class="Ring (strict)"(error in=w523, "Strings []"=w524) -> (error out=w522:errorcluster)  [unwired: 1 in, 1 out]
          }
        }
        n233 = call "SubVI_Example_GetFramerate.vi"(".NET (Reference)"=w420, "Error In"=w435) -> ("Min"=w427:dbl, "Max"=w426:dbl, "error out"=w434:errorcluster)  [unwired: 9 in, 2 out]
        "MaxFps" <- w426
        "MinFps" <- w427
        n234 = call "SubVI_Example_Timing.vi"(".NET (Reference)"=w420, "Pixelclock"=w474, "Exposure time"=w473, "Framerate"=w472, "Error In"=w434) -> ("Pixelclock"=w419:i32, "Exposure time"=w430:dbl, "Framerate"=w429:dbl, "Error Out"=w418:errorcluster)  [unwired: 7 in]
        n235 = property on="Pixelclock" class="Ring (strict)"(error in=w418) -> (error out=w416:errorcluster, "Strings []"=w417:string[])  [unwired: 1 in, 1 out]
        n236 = while {
          tunnel: w419 -> [w492]
          tunnel: w417 -> [w497]
          tunnel: w416 -> [w491]
          tunnel: [w492] -> w415
          tunnel: [w491] -> w414
          i -> [w496]
          stop <- w493 stop-if-true
          n237 = Number To Decimal String(number=w492) -> (decimal integer string=w494:string)  [unwired: 1 in]
          n238 = Index Array(array=w497, index=w496) -> (element=w495:string)
          n239 = Equal?(x=w494, y=w495) -> (x = y?=w493:bool)
        }
        n240 = property on="Pixelclock" class="Ring (strict)"(error in=w414, "Value"=w415) -> (error out=w413:errorcluster)  [unwired: 1 in, 1 out]
        n241 = property on="Framerate" class="DigNum (strict)"(error in=w413, "Value"=w429, "Maximum"=w426, "Minimum"=w427) -> (error out=w422:errorcluster)  [unwired: 1 in, 1 out]
        n242 = call "SubVI_Example_GetExposure.vi"(".NET (Reference)"=w420, "Error In"=w422) -> ("Inc"=w423:dbl, "Min"=w424:dbl, "Max"=w425:dbl, "Error out"=w421:errorcluster)  [unwired: 9 in, 1 out]
        n243 = property on="Exposure" class="Slide (strict)"(error in=w421, "Value"=w430, "Scale.Increment"=w423, "Scale.Maximum"=w425, "Scale.Minimum"=w424) -> (error out=w428:errorcluster)  [unwired: 1 in, 1 out]
        n244 = call "SubVI_Example_MemoryAllocation.vi"(".NET (Reference)"=w420, "Error In"=w428) -> ("Bits/Pixel 2"=→"Bits/Pixel":i32, "Width"=→"Width":i32, "Serial Number"=→"Serial Number":string, "Height"=→"Height":i32, "Error Out"=w451:errorcluster)  [unwired: 13 in]
      }
      frame "Start live" {
        # "Has acquisition started?"
        # "Start Acquisition"
        n245 = property class="Camera"(reference=w552, error in=w553) -> (error out=w562:errorcluster, "Acquisition"=w561:refnum<k24>)  [unwired: 1 out]
        n246 = invoke class="Acquisition" method="HasStarted"(reference=w561, error in=w562) -> (reference out=w557:refnum<k24>, error out=w556:errorcluster, "HasStarted"=w555:i32, "bValue"=w560:bool)  [unwired: 2 in]
        n247 = control-ref of="Start Live"() -> (w549:refnum<vi>)
        n248 = control-ref of="Load Parameter"() -> (w546:refnum<vi>)
        n249 = control-ref of="Stop Live"() -> (w544:refnum<vi>)
        n250 = invoke class="Acquisition" method="ToString"(reference=w557, error in=w556) -> (error out=w559:errorcluster, "ToString"=w558:string)  [unwired: 1 in, 1 out]
        n251 = property class="Bool"(reference=w549, "Disabled"=u8 2 ("Deaktiviert")) -> (reference out=w538:refnum<vi>, error out=w537:errorcluster)  [unwired: 1 in]
        n252 = property class="Bool"(reference=w546, "Disabled"=u8 2 ("Deaktiviert")) -> (reference out=w540:refnum<vi>, error out=w539:errorcluster)  [unwired: 1 in]
        n253 = property class="Bool"(reference=w544, "Disabled"=u8 0 ("Deaktiviert")) -> (reference out=w542:refnum<vi>, error out=w541:errorcluster)  [unwired: 1 in]
        n254 = call "Error_Handling.vi"("Error Code"=w555, "Error String"=w558, "Error In"=w559) -> ("Error Out"=w554:errorcluster)  [unwired: 8 in]
        n255 = Close Reference(reference=w538, error in (no error)=w537) -> ()  [unwired: 1 out]
        n256 = Close Reference(reference=w540, error in (no error)=w539) -> ()  [unwired: 1 out]
        n257 = Close Reference(reference=w542, error in (no error)=w541) -> ()  [unwired: 1 out]
        n258 = case shown="False" w560 {
          tunnel: [w565 w575] -> w550
          tunnel: w554 -> [w571 w575]
          tunnel: w552 -> [w570 w574]
          tunnel: [w570 w574] -> w536
          frame False {
            w563 = 1 items=["IS_DONT_WAIT", "IS_WAIT"] ("Wait")
            n259 = property class="Camera"(reference=w570, error in=w571) -> (error out=w572:errorcluster, "Acquisition"=w573:refnum<k24>)  [unwired: 1 out]
            n260 = invoke class="Acquisition" method="Capture"(reference=w573, error in=w572, "param"=w563) -> (reference out=w566:refnum<k24>, error out=w567:errorcluster, "Capture"=w564:i32)  [unwired: 1 in, 1 out]
            n261 = invoke class="Acquisition" method="ToString"(reference=w566, error in=w567) -> (error out=w569:errorcluster, "ToString"=w568:string)  [unwired: 1 in, 1 out]
            n262 = call "Error_Handling.vi"("Error Code"=w564, "Error String"=w568, "Error In"=w569) -> ("Error Out"=w565:errorcluster)  [unwired: 8 in]
          }
          frame True {
          }
        }
      }
    }
    n263 = call "SubVI_Example_SyncEventLoop.vi"("Error In"=w47, "use sync"=w31, ".NET (Reference)"=w30) -> ("Error Out"=w45:errorcluster, "Synchronize (ms)"=w46:dbl)  [unwired: 7 in]
    "Error Out" <- w45
    n264 = Wait Until Next ms Multiple(millisecond multiple=w46) -> ()  [unwired: 1 out]
  }
